vi "GetRazdelitel(SubVI).vi"() -> (0 "comm?":bool)   [LabVIEW 2017]
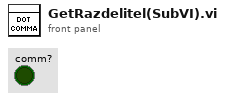
[diagram p1: front panel]
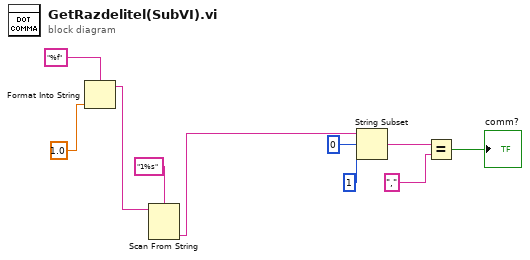
[diagram p0: block diagram]
diagram:
  n1 = Format Into String(format string="%f" ("initial string"), 1.0 ("input 1")) -> (resulting string=w10:string)  [unwired: 2 in, 1 out]
  n2 = Scan From String(format string="1%s", input string=w10) -> (output 1=w6:string)  [unwired: 3 in, 3 out]
  n3 = String Subset(string=w6, offset (0)=0, length (rest)=1 ("length (rest)")) -> (substring=w2:string)
  n4 = Equal?(x=w2, y="," ("format string")) -> (x = y?=→"comm?":bool)
